vi "Calibration_Test.vi"() -> ()   [LabVIEW 2021]
uses:
  C:/Users/User/Documents/CB III control files/Thorlabs.MotionControl.Controls.dll
  CB III control files/Thorlabs.MotionControl.Controls.dll
  C:/Users/User/Documents/CB III control files/ThorLabs.MotionControl.Benchtop.DCServoCLI.dll
  CB III control files/ThorLabs.MotionControl.Benchtop.DCServoCLI.dll
  C:/Users/User/Documents/CB III control files/ThorLabs.MotionControl.KCube.DCServoCLI.dll
  CB III control files/ThorLabs.MotionControl.KCube.DCServoCLI.dll
  C:/Users/User/Documents/CB III control files/Thorlabs.MotionControl.IntegratedStepperMotorsCLI.dll
  CB III control files/Thorlabs.MotionControl.IntegratedStepperMotorsCLI.dll
  <vilib>/Utility/file.llb/Write Delimited Spreadsheet (DBL).vi
  <vilib>/Utility/file.llb/Read Delimited Spreadsheet (DBL).vi
  Global_Stop.vi
  <vilib>/ptbypt/NI_PtbyPt.lvlib
panel:
  out "Lumedica report 2":string
  in  "saveing method 2":string(combo)="SaveQueueImages"
  out "OCT ON":bool=TRUE
  out "Lumedica report":string
  in  "saveing method":string(combo)="SaveQueueImages"
  in  "?":bool
  out "OCT imaging position":dbl[](array[numeric])
  in  "?":bool
  in  "?":bool
  out "all pilot points":dbl[][](array[numeric])
  out "X-stage Control":refnum<k24>
  out "X stage properties":refnum<k24>
  in  "LongTravelStageControl":refnum<k24>(container)
  out "Zero Position":dbl[](array[numeric])
  out "Drill-Z-stage Control":refnum<k24>
  out "OCT-Z-stage-control":refnum<k24>
  out "Y-stage Control":refnum<k24>
  out "Y-stage properties":refnum<k24>
  out "Driller-Z-stage-Properties":refnum<k24>
  out "OCT-Z stage-properites":refnum<k24>
  in  "Trajectory":dbl[][](array[numeric])
  out "Velocity":T1(graph)
  out "position":T1(graph)
  in  "Driller Z- stage":refnum<k24>(container)
  in  "Y stage":refnum<k24>(container)
  in  "OCT Z-stage":refnum<k24>(container)
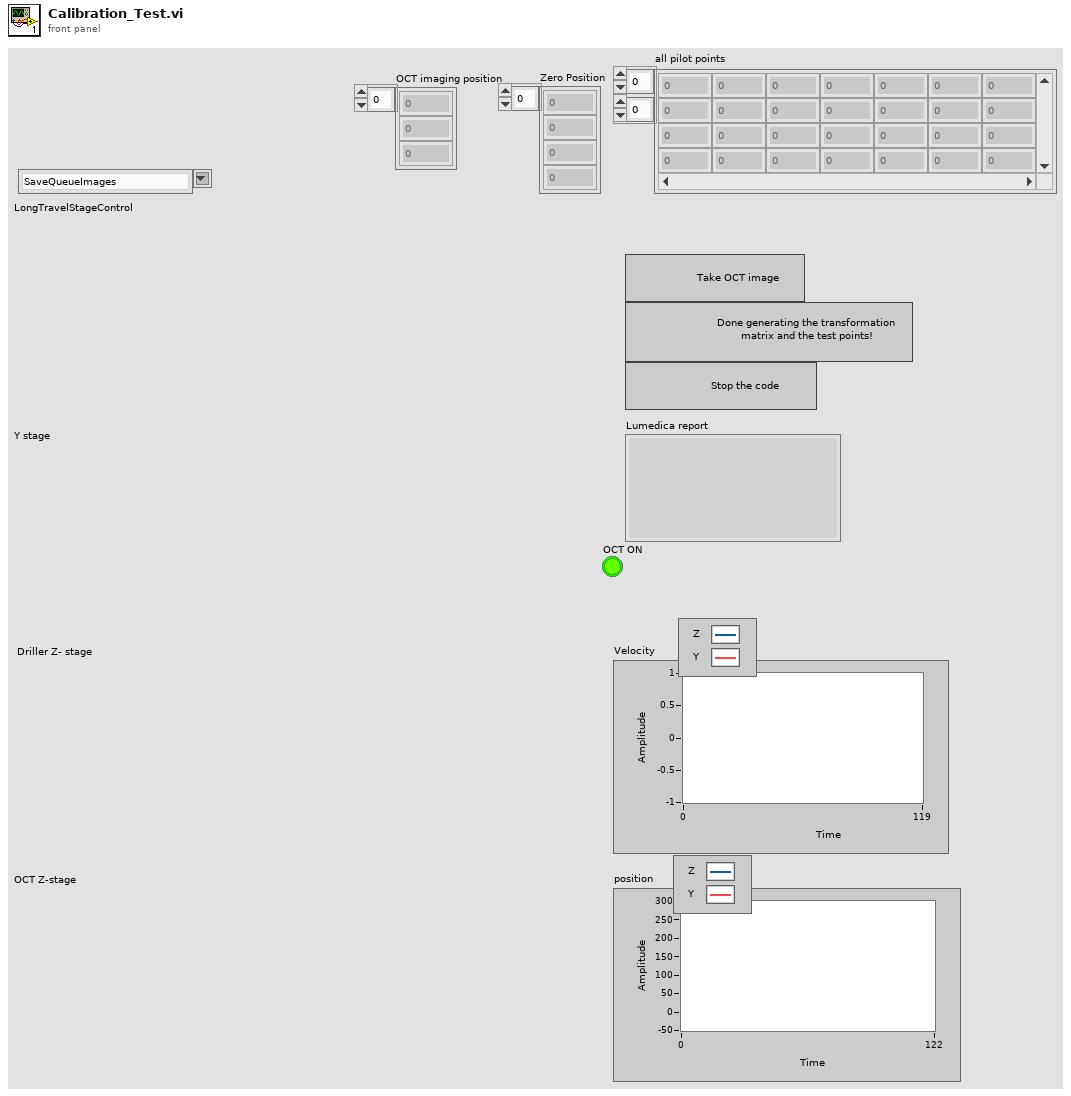
[diagram p1: front panel]
types:
  T1 = cluster{"[0]":dbl, "[1]":dbl, "[2]":dbl, "[3]":dbl, "[4]":dbl, "[5]":dbl, "[6]":dbl, "[7]":dbl, "[8]":dbl}
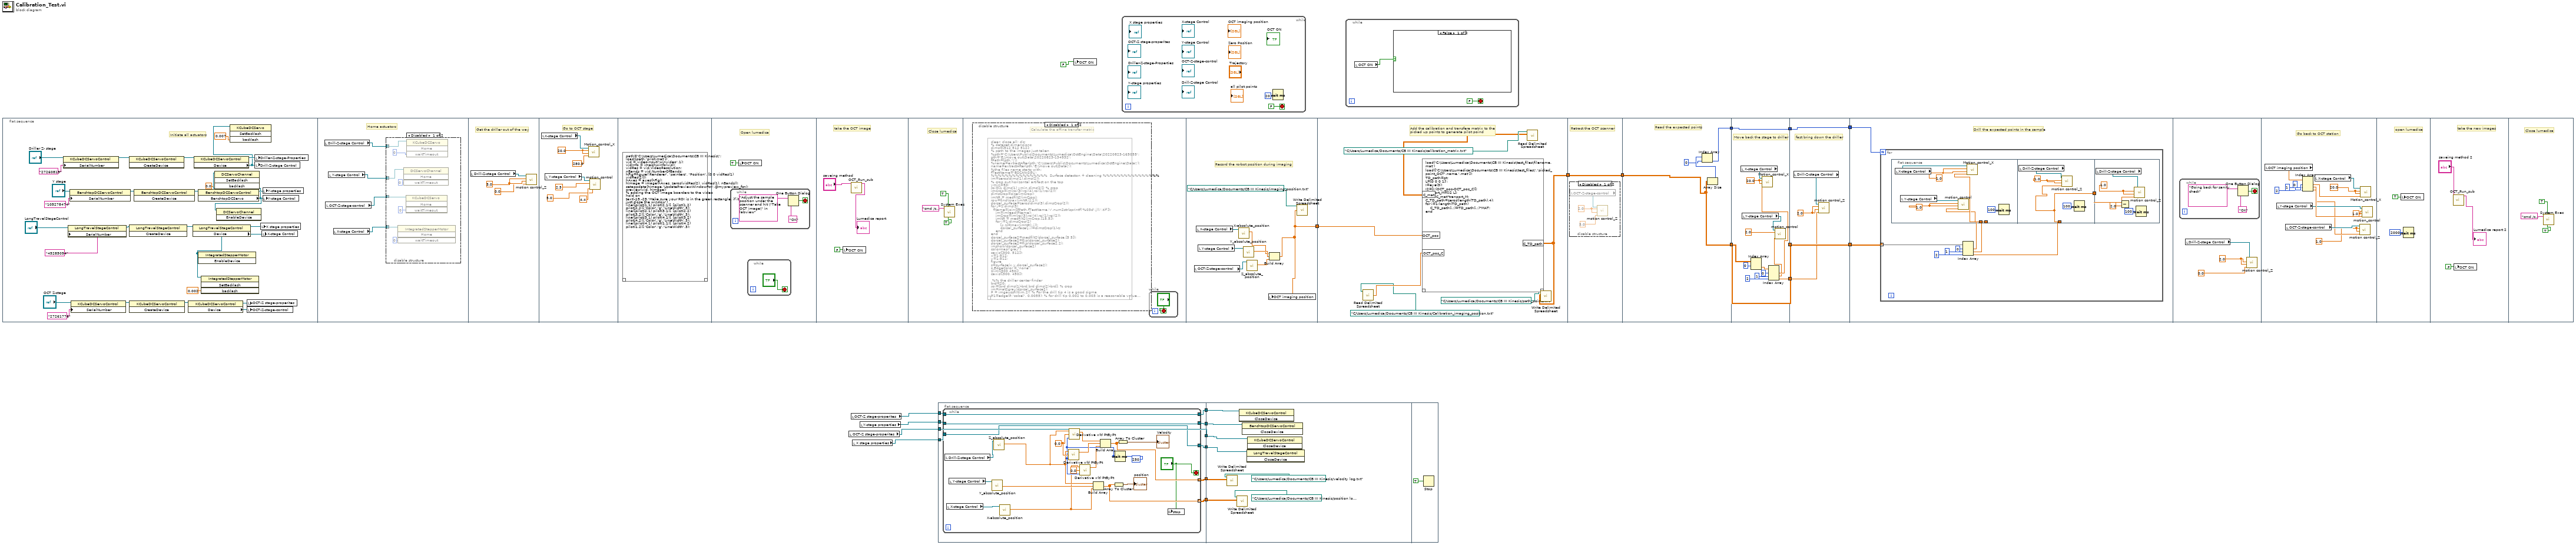
[diagram p0: block diagram]
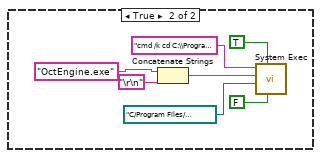
[diagram p2: hidden frame]
diagram:
  n1 = flat-sequence {
    tunnel: [w83] -> w10
    tunnel: w10 -> [w95]
    tunnel: [w91] -> w1
    tunnel: [w98] -> w2
    tunnel: w1 -> [w98]
    tunnel: [w103] -> w7
    tunnel: [w102] -> w5
    tunnel: w2 -> [w102]
    tunnel: w7 -> [w119]
    tunnel: [w119] -> w6
    tunnel: w5 -> [w114]
    tunnel: [w114] -> w4
    tunnel: [w106] -> w3
    tunnel: w6 -> [w124]
    tunnel: [w124] -> w9
    tunnel: w4 -> [w123]
    tunnel: [w123] -> w8
    tunnel: w3 -> [w120]
    tunnel: w9 -> [w126]
    tunnel: w8 -> [w125]
    frame #0 {
      # "Initiate all actuators"
      n2 = property class="KCubeDCServoControl"(reference="Driller Z- stage", "SerialNumber"="27260819") -> (reference out=w43:refnum<k24>)  [unwired: 1 in, 1 out]
      n3 = property class="LongTravelStageControl"(reference="LongTravelStageControl", "SerialNumber"="45285094") -> (reference out=w28:refnum<k24>)  [unwired: 1 in, 1 out]
      n4 = property class="BenchtopDCServoControl"(reference="Y stage", "SerialNumber"="105278474") -> (reference out=w40:refnum<k24>)  [unwired: 1 in, 1 out]
      n5 = property class="KCubeDCServoControl"(reference="OCT Z-stage", "SerialNumber"="27261776") -> (reference out=w48:refnum<k24>)  [unwired: 1 in, 1 out]
      n6 = invoke class="KCubeDCServoControl" method="CreateDevice"(reference=w43) -> (reference out=w38:refnum<k24>)  [unwired: 2 in, 2 out]
      n7 = invoke class="LongTravelStageControl" method="CreateDevice"(reference=w28) -> (reference out=w27:refnum<k24>)  [unwired: 2 in, 2 out]
      n8 = invoke class="KCubeDCServoControl" method="CreateDevice"(reference=w48) -> (reference out=w45:refnum<k24>)  [unwired: 2 in, 2 out]
      n9 = invoke class="BenchtopDCServoControl" method="CreateDevice"(reference=w40) -> (reference out=w37:refnum<k24>)  [unwired: 2 in, 2 out]
      n10 = property class="KCubeDCServoControl"(reference=w45) -> (reference out=w36:refnum<k24>, "Device"=w33:refnum<k24>)  [unwired: 1 in, 1 out]
      n11 = property class="LongTravelStageControl"(reference=w27) -> (reference out=w26:refnum<k24>, "Device"=w25:refnum<k24>)  [unwired: 1 in, 1 out]
      n12 = property class="KCubeDCServoControl"(reference=w38) -> (reference out=w35:refnum<k24>, "Device"=w31:refnum<k24>)  [unwired: 1 in, 1 out]
      n13 = property class="BenchtopDCServoControl"(reference=w37) -> (reference out=w34:refnum<k24>, "BenchtopDCServo"=w23:refnum<k24>)  [unwired: 1 in, 1 out]
      n14 = invoke class="IntegratedStepperMotor" method="EnableDevice"(reference=w25) -> ()  [unwired: 2 in, 3 out]
      n15 = invoke class="IntegratedStepperMotor" method="SetBacklash"(reference=w25, "backlash"=0.002) -> ()  [unwired: 2 in, 4 out]
      n16 = invoke class="DCServoChannel" method="SetBacklash"(reference=w23, "backlash"=0.0) -> ()  [unwired: 2 in, 4 out]
      n17 = invoke class="DCServoChannel" method="EnableDevice"(reference=w23) -> ()  [unwired: 2 in, 3 out]
      n18 = invoke class="KCubeDCServo" method="SetBacklash"(reference=w31, "backlash"=0.007) -> ()  [unwired: 2 in, 4 out]
      n19 = local write "OCT-Z stage-properites"(w36) -> ()
      n20 = local write "OCT-Z-stage-control"(w33) -> ()
      n21 = local write "Driller-Z-stage-Properties"(w35) -> ()
      n22 = local write "Drill-Z-stage Control"(w31) -> ()
      n23 = local write "X stage properties"(w26) -> ()
      n24 = local write "X-stage Control"(w25) -> ()
      n25 = local write "Y-stage properties"(w34) -> ()
      n26 = local write "Y-stage Control"(w23) -> ()
    }
    frame #1 {
      # "Home actuators"
      n27 = local read "Drill-Z-stage Control"() -> (w52:refnum<k24>)
      n28 = local read "OCT-Z-stage-control"() -> (w50:refnum<k24>)
      n29 = local read "Y-stage Control"() -> (w51:refnum<k24>)
      n30 = local read "X-stage Control"() -> (w49:refnum<k24>)
      n31 = disable-structure shown="Disabled" {
        disable-tunnel: w51 -> [w60 _]
        disable-tunnel: w52 -> [w58 _]
        disable-tunnel: w50 -> [w56 _]
        disable-tunnel: w49 -> [w54 _]
        frame Disabled {
          n32 = invoke class="IntegratedStepperMotor" method="Home"(reference=w54, "waitTimeout"=0) -> ()  [unwired: 2 in, 4 out]
          n33 = invoke class="DCServoChannel" method="Home"(reference=w60, "waitTimeout"=0) -> ()  [unwired: 2 in, 4 out]
          n34 = invoke class="KCubeDCServo" method="Home"(reference=w56, "waitTimeout"=0) -> ()  [unwired: 2 in, 4 out]
          n35 = invoke class="KCubeDCServo" method="Home"(reference=w58, "waitTimeout"=0) -> ()  [unwired: 2 in, 4 out]
        }
        frame Enabled {
        }
      }
    }
    frame #2 {
      w62 = 3.0 ("maxVelocity")
      # "Get the driller out of the way"
      n36 = local read "Drill-Z-stage Control"() -> (w63:refnum<k24>)
      n37 = call "motion control_Z.vi"("position"=0.0, "acceleration"=w62, "maxVelocity"=w62, ".NET Refnum in"=w63) -> ()  [unwired: 1 in, 1 out]
    }
    frame #3 {
      w66 = 20.0 ("maxVelocity")
      # "Go to OCT stage"
      n38 = local read "X-stage Control"() -> (w70:refnum<k24>)
      n39 = local read "Y-stage Control"() -> (w69:refnum<k24>)
      n40 = call "Motion_control_X.vi"(".NET Refnum in"=w70, "maxVelocity"=w66, "acceleration"=w66, "position"=280.0) -> ()  [unwired: 6 in, 1 out]
      n41 = call "motion_control.vi"("position"=4.4, "acceleration"=5.0, "maxVelocity"=2.5, ".NET Refnum in"=w69) -> ()  [unwired: 1 in, 1 out]
    }
    frame #4 {
      n42 = script code="path='C:\\Users\\Lumedica\\Documents\\CB III Kinesis\\';\nload([path,'pilot.mat'])\nvid = videoinput('winvideo',1);\nvidInfo = imaqhwinfo(vid);\nvidRes = vid.VideoResolution;\nnBands = vid.NumberOfBands; \nhFig=figure('Renderer', 'painters', 'Position', [0 0 vidRes(1) vidRes(2)]);\nhAxes = axes(hFig);\nhImage = image(hAxes, zeros(vidRes(2), vidRes(1), nBands)); \nsetappdata(hImage,'UpdatePreviewWindowFcn',@mypreview_fcn);\npreview(vid, hImage); \n% adding the OCT image boarders to the video\nhold on\ntext(-15,-25,'Make sure your ROI is in the green rectangle. if it is, just close the window')\nline([pilot(1,1) pilot(2,1)], [pilot(1,2) pilot(2,2)],'Color','g','LineWidth',3);\nline([pilot(2,1) pilot(3,1)], [pilot(2,2) pilot(3,2)],'Color','g','LineWidth',3);\nline([pilot(3,1) pilot(4,1)], [pilot(3,2) pilot(4,2)],'Color','g','LineWidth',3);\nline([pilot(4,1) pilot(1,1)], [pilot(4,2) pilot(1,2)],'Color','g','LineWidth',3);"() -> ()  [unwired: 1 in, 1 out]
    }
    frame #5 {
      # "Open lumedica"
      n43 = while {
        stop <- w75 stop-if-true
        n44 = One Button Dialog(message="Adjust the sample position under the scanner and hit \"Take OCT image\" in labview", button name ("OK")="OK") -> (true=w75:bool)
      }
      n45 = local write "OCT ON"(TRUE ("OCT ON")) -> ()
      n46 = while {
        stop <- "?" stop-if-true
      }
    }
    frame #6 {
      # "take the OCT image"
      n47 = local write "OCT ON"(FALSE ("OCT ON")) -> ()
      n48 = call "OCT_Run_sub.vi"("saveing method"="saveing method") -> ("Lumedica report"=→"Lumedica report":string)  [unwired: 10 in]
    }
    frame #7 {
      # "Close lumedica"
      n49 = call <vilib>:"System Exec.vi"("run minimized? (F)"=TRUE, "wait until completion? (T)"=TRUE, "command line"="cmd /c taskkill /IM OctEngine.exe") -> ()  [unwired: 5 in, 4 out]
    }
    frame #8 {
      n50 = disable-structure shown="Disabled" {
        frame Disabled {
          # "Calculate the affine transfer matrix"
          n51 = script code="clear; close all; clc;\n% dataset dimensions\ndims=[512 512 512]; \n% path to the images just taken\n%pth='C:\\Users\\Public\\Documents\\Lumedica\\OctEngine\\Data\\20220823-165055';\npth='E:\\move out\\Data\\20220823-134932';\nfPath=[pth,'\\'];\n%name=extractAfter(pth,'C:\\Users\\Public\\Documents\\Lumedica\\OctEngine\\Data\\');\nname=extractAfter(pth,'E:\\move out\\Data\\');\n%the files name starts with:\nfTestName='BSCAN-SGL';\n%%%%%%%%%%%%%%%%  Surface detecton + cleaning %%%%%%%%%%%%%%%%\nim=zeros(dims(1),dims(2)); \n% crop out horizontal artifact on the top\nymin=50;\nroi=[1 dims(1) ymin dims(2)]; % crop\nimCrop=im(roi(3):roi(4),roi(1):roi(2));\ndimsCrop=size(imCrop);\nimNR = medfilt2(imCrop);\nrow=find(max(imNR,[],1));\ndorsal_surface=zeros(dims(3),dimsCrop(2));\nfor j=1:dims(3)\n  fName=join([fPath,fTestName,'-',num2str(sprintf('%03d',j)),'.tif']);\n    im=imread(fName);\n    imCrop=im(roi(3):roi(4),roi(1):roi(2));\n    imNR = medfilt2(imCrop,[15,5]);\n    for i=1:dimsCrop(2)\n        [x,z]=max(imNR(:,i));\n        dorsal_surface(j,i)=dimsCrop(1)-z;\n    end\nend\ndorsal_surface2=medfilt2(dorsal_surface,[5 5]);\ndorsal_surface2=flip(dorsal_surface2);\ndorsal_surface2=flip(dorsal_surface2,2);\nimshow(dorsal_surface2)\ncolormap('gray')\ncaxis([300, 512]);\nx=1:512;\ny=1:512;\nfigure\ns=surface(x,y,dorsal_surface2);\ns.EdgeColor = 'none';\nzlim([300 450])\ncaxis([300, 450]);\n\n %% the driller center finder\nbrd=20;\nroi=[brd dims(1)-brd brd dims(2)-brd]; % crop\nim=mat2gray(dorsal_surface2);\nP = imgaussfilt(im,2); % For the drill tip 4 is a good sigma\nP1=edge(P,'sobel', 0.0055); % for drill tip 0.002 to 0.003 is a reasonable value\nse10 = strel('disk',2);\nP2=imdilate(P1,se10);\nP3 = imfill(P2,'holes');\nfigure\nsubplot(1,4,1)\nimshow(P1)\nsubplot(1,4,2)\nimshow(P2)\nsubplot(1,4,3)\nimshow(P3)\nP3=P3(roi(3):roi(4),roi(1):roi(2));\n[centers, radii, metric] = imfindcircles(P3,[7 45]);\ncenters=round(centers)+brd;\nsubplot(1,4,4)\n imshow(dorsal_surface2);\n caxis([300, 512]);\nviscircles(centers,radii,'LineWidth',0.4);\n% Sort the centers\ncenters=sortrows(centers,1); % right to left\ncenters=sortrows(centers,2); % sort centers top to bottom\nsave('Detected_circles5.mat','centers','radii'); \n% add their depth to them\ndorsal_surface3=medfilt2(dorsal_surface2,[5 5]);\nfor i=1:length(centers)\n    depth(i)=dorsal_surface3(centers(i,2),centers(i,1));\nend\n%% Generating the transformation matrix\n%/////////////////////DO NOT RUN DURING SANITY CHECK!\\\\\\\\\\\\\\\\\\\\\\\\\\\\\\\\\\\\\\\\\n%Generating world data\nfigure\n imshow(dorsal_surface2);\n caxis([300, 512]);\nviscircles(centers,radii,'LineWidth',0.4);\npath='C:\\Users\\User\\Documents\\CB III Kinesis\\Generated_calibration_points.txt';\npoints=importdata(path)';     %rows are each points columns are from left to right: X Y Z 1\n%Genrate OCT points in the same order\ncenters_all=[centers depth' ones(length(depth),1)];\nOCT2World=centers_all\\points; % left side multiply the transformation matrix\n[X,Y]=getpts; %press inter when done selecting\nC=[X,Y];\nfor o=1:length(X)\nviscircles([X(o),Y(o)],7.5,'LineWidth',0.4,'Color','b')\npt(o,:)=[round(X(o));round(Y(o));dorsal_surface2(round(Y(o)),round(X(o)));1]';\nW(o,:)=pt(o,:)*OCT2World;\nend\nsave(['picked_point_OCT11',name,'.mat'],'pt')\nsave(['picked_point_real',name,'.mat'],'W')\nsave(['previouse circles',name,'.mat'],'centers','radii')\nPname='C:\\Users\\User\\Documents\\CB III Kinesis\\test_points.txt';\nCLname='C:\\Users\\User\\Documents\\CB III Kinesis\\calibration_matric.txt';\nwritematrix(W,Pname,'Delimiter','tab')  % save the test point coordinates for drilling\nwritematrix(OCT2World,CLname,'Delimiter','tab') % save the calibration matrix"() -> ()  [unwired: 1 in, 1 out]
        }
        frame Enabled {
        }
      }
      n52 = while {
        stop <- "?" stop-if-true
      }
    }
    frame #9 {
      # "Record the rorbot position during imaging"
      n53 = local read "OCT-Z-stage-control"() -> (w84:refnum<k24>)
      n54 = local read "X-stage Control"() -> (w85:refnum<k24>)
      n55 = local read "Y-stage Control"() -> (w86:refnum<k24>)
      n56 = call "X-absolute_position.vi"(".NET Refnum in"=w85) -> ("Numeric"=w88:dbl)  [unwired: 9 in, 1 out]
      n57 = call "Y_absolute_position.vi"(".NET Refnum in"=w86) -> ("Numeric"=w89:dbl)  [unwired: 9 in, 1 out]
      n58 = call "Z_absolute_position.vi"(".NET Refnum in"=w84) -> ("Numeric"=w90:dbl)  [unwired: 9 in, 1 out]
      n59 = Build Array(w88, w89, w90) -> (w83:dbl[])
      n60 = local write "OCT imaging position"(w83) -> ()
      n61 = call-poly <vilib>:"Write Delimited Spreadsheet.vi"("file path (dialog if empty)"=path "C:/Users/Lumedica/Documents/CB III Kinesis/imaging_position.txt", "1D data"=w83) -> ()  [unwired: 12 in, 2 out]
    }
    frame #10 {
      # "Add the calibration and transfere matrix to the \npicked up points to generate pilot poind"
      n62 = call-poly <vilib>:"Read Delimited Spreadsheet.vi"("file path (dialog if empty)"=path "C:/Users/Lumedica/Documents/CB III Kinesis/Calibration_imaging_position.txt") -> ("first row"=w94:dbl[])  [unwired: 9 in, 5 out]
      n63 = call-poly <vilib>:"Read Delimited Spreadsheet.vi"("file path (dialog if empty)"=path "C:/Users/Lumedica/Documents/CB III Kinesis/calibration_matrix.txt") -> ("all rows"=w96:dbl[][])  [unwired: 9 in, 5 out]
      n64 = script code="load('C:\\Users\\Lumedica\\Documents\\CB III Kinesis\\test_files\\filename.mat')\nload(['C:\\Users\\Lumedica\\Documents\\CB III Kinesis\\test_files\\','picked_point_OCT',name,'.mat']);\nTD_path=pt;\nL=[0 0 0 1]';\nI=eye(3);\nI2=[I;(OCT_pos-OCT_pos_C)];\ntranport_M=[I2 L];\nMAT=C_mat*tranport_M;\nC_TD_path=zeros(length(TD_path),4);\nfor i=1:length(TD_path)\n    C_TD_path(i,:)=TD_path(i,:)*MAT;\nend"("OCT_pos_C"=w94, "OCT_pos"=w95, "C_mat"=w96) -> ("C_TD_path"=w91:dbl[][])  [unwired: 1 in, 1 out]
      n65 = call-poly <vilib>:"Write Delimited Spreadsheet.vi"("file path (dialog if empty)"=path "C:/Users/Lumedica/Documents/CB III Kinesis/path_points.txt", "2D data"=w91) -> ()  [unwired: 12 in, 2 out]
    }
    frame #11 {
      # "Retract the OCT scanner"
      n66 = disable-structure shown="Disabled" {
        frame Disabled {
          w99 = 2.0 ("maxVelocity")
          n67 = local read "OCT-Z-stage-control"() -> (w101:refnum<k24>)
          n68 = call "motion control_Z.vi"("position"=5.0, "acceleration"=w99, "maxVelocity"=w99, ".NET Refnum in"=w101) -> ()  [unwired: 1 in, 1 out]
        }
        frame Enabled {
        }
      }
    }
    frame #12 {
      # "Read the expected points"
      n69 = Array Size(array=w102) -> (size(s)=w105:i32[])
      n70 = Index Array(array=w105, index=0) -> (element=w103:i32)
    }
    frame #13 {
      w115 = 20.0 ("maxVelocity")
      w116 = 2.0 ("maxVelocity")
      # "Move back the stage to driller"
      n71 = local read "X-stage Control"() -> (w117:refnum<k24>)
      n72 = local read "Y-stage Control"() -> (w118:refnum<k24>)
      n73 = Index Array(array=w114, index (row)=0) -> (element=w112:dbl[])  [unwired: 1 in]
      n74 = Index Array(array=w112, index #1=0 ("index"), index #2=1 ("index"), index #3=2 ("index")) -> (element #1=w108:dbl, element #2=w107:dbl, element #3=w106:dbl)
      n75 = call "Motion_control_X.vi"(".NET Refnum in"=w117, "maxVelocity"=w115, "acceleration"=w115, "position"=w108) -> ()  [unwired: 6 in, 1 out]
      n76 = call "motion_control.vi"("position"=w107, "acceleration"=w116, "maxVelocity"=w116, ".NET Refnum in"=w118) -> ()  [unwired: 1 in, 1 out]
    }
    frame #14 {
      w121 = 2.0 ("acceleration")
      # "fast bring down the driller"
      n77 = local read "Drill-Z-stage Control"() -> (w122:refnum<k24>)
      n78 = call "motion control_Z.vi"("position"=w120, "acceleration"=w121, "maxVelocity"=w121, ".NET Refnum in"=w122) -> ()  [unwired: 1 in, 1 out]
    }
    frame #15 {
      # "Drill the expected points in the sample"
      n79 = for {
        N: w126 -> [_]
        tunnel: w125 -> [w134] mode=indexing
        n80 = flat-sequence {
          tunnel: w130 -> [w136]
          tunnel: w129 -> [w135]
          tunnel: w128 -> [w142]
          tunnel: [w142] -> w127
          tunnel: w127 -> [w146]
          frame #0 {
            w137 = 1.0 ("maxVelocity")
            w138 = 1.0 ("maxVelocity")
            n81 = local read "X-stage Control"() -> (w139:refnum<k24>)
            n82 = local read "Y-stage Control"() -> (w140:refnum<k24>)
            n83 = call "motion_control.vi"("position"=w135, "acceleration"=w137, "maxVelocity"=w137, ".NET Refnum in"=w140) -> ()  [unwired: 1 in, 1 out]
            n84 = call "Motion_control_X.vi"(".NET Refnum in"=w139, "maxVelocity"=w138, "acceleration"=w138, "position"=w136) -> ()  [unwired: 6 in, 1 out]
            n85 = Wait (ms)(milliseconds to wait=u32 100) -> ()  [unwired: 1 out]
          }
          frame #1 {
            w144 = 1.0 ("maxVelocity")
            n86 = local read "Drill-Z-stage Control"() -> (w145:refnum<k24>)
            n87 = call "motion control_Z.vi"("position"=w142, "acceleration"=w144, "maxVelocity"=w144, ".NET Refnum in"=w145) -> ()  [unwired: 1 in, 1 out]
            n88 = Wait (ms)(milliseconds to wait=u32 100) -> ()  [unwired: 1 out]
          }
          frame #2 {
            w150 = 1.0 ("maxVelocity")
            n89 = local read "Drill-Z-stage Control"() -> (w151:refnum<k24>)
            n90 = Subtract(x=w146, y=2.0) -> (x-y=w148:dbl)
            n91 = call "motion control_Z.vi"("position"=w148, "acceleration"=w150, "maxVelocity"=w150, ".NET Refnum in"=w151) -> ()  [unwired: 1 in, 1 out]
            n92 = Wait (ms)(milliseconds to wait=u32 100) -> ()  [unwired: 1 out]
          }
        }
        n93 = Index Array(array=w134, index #1=0 ("index"), index #2=1 ("index"), index #3=2 ("index")) -> (element #1=w130:dbl, element #2=w129:dbl, element #3=w128:dbl)
      }
    }
    frame #16 {
      w152 = 2.0 ("maxVelocity")
      n94 = while {
        stop <- w157 stop-if-true
        n95 = One Button Dialog(message="Going back for sanity check", button name ("OK")="OK") -> (true=w157:bool)
      }
      n96 = local read "Drill-Z-stage Control"() -> (w154:refnum<k24>)
      n97 = call "motion control_Z.vi"("position"=0.0, "acceleration"=w152, "maxVelocity"=w152, ".NET Refnum in"=w154) -> ()  [unwired: 1 in, 1 out]
    }
    frame #17 {
      w158 = 1.0 ("maxVelocity")
      w162 = 1.0 ("acceleration")
      w165 = 20.0 ("maxVelocity")
      # "Go back to OCT station"
      n98 = local read "OCT imaging position"() -> (w167:dbl[])
      n99 = local read "Y-stage Control"() -> (w161:refnum<k24>)
      n100 = local read "OCT-Z-stage-control"() -> (w160:refnum<k24>)
      n101 = Index Array(array=w167, index #1=0 ("index"), index #2=1 ("index"), index #3=2 ("index")) -> (element #1=w164:dbl, element #2=w163:dbl, element #3=w159:dbl)
      n102 = local read "X-stage Control"() -> (w166:refnum<k24>)
      n103 = call "motion control_Z.vi"("position"=w159, "acceleration"=w158, "maxVelocity"=w158, ".NET Refnum in"=w160) -> ()  [unwired: 1 in, 1 out]
      n104 = call "Motion_control_X.vi"(".NET Refnum in"=w166, "maxVelocity"=w165, "acceleration"=w165, "position"=w164) -> ()  [unwired: 6 in, 1 out]
      n105 = call "motion_control.vi"("position"=w163, "acceleration"=w162, "maxVelocity"=w162, ".NET Refnum in"=w161) -> ()  [unwired: 1 in, 1 out]
    }
    frame #18 {
      # "open lumedica"
      n106 = local write "OCT ON"(TRUE ("OCT ON")) -> ()
      n107 = Wait (ms)(milliseconds to wait=u32 2000) -> ()  [unwired: 1 out]
    }
    frame #19 {
      # "take the new images"
      n108 = call "OCT_Run_sub.vi"("saveing method"="saveing method 2") -> ("Lumedica report"=→"Lumedica report 2":string)  [unwired: 10 in]
      n109 = local write "OCT ON"(FALSE ("OCT ON")) -> ()
    }
    frame #20 {
      # "Close lumedica"
      n110 = call <vilib>:"System Exec.vi"("run minimized? (F)"=TRUE, "wait until completion? (T)"=TRUE, "command line"="cmd /c taskkill /IM OctEngine.exe") -> ()  [unwired: 5 in, 4 out]
    }
  }
  n111 = local read "OCT-Z stage-properites"() -> (w16:refnum<k24>)
  n112 = local read "OCT-Z stage-properites"() -> (w21:refnum<k24>)
  n113 = local read "X stage properties"() -> (w13:refnum<k24>)
  n114 = local read "Y-stage properties"() -> (w20:refnum<k24>)
  n115 = flat-sequence {
    tunnel: w21 -> [w185]
    tunnel: w20 -> [w184]
    tunnel: [w183] -> w19
    tunnel: [w187] -> w18
    tunnel: [w186] -> w17
    tunnel: w16 -> [w183]
    tunnel: [w182] -> w15
    tunnel: [w181] -> w14
    tunnel: w13 -> [w180]
    tunnel: [w179] -> w12
    tunnel: w19 -> [w213]
    tunnel: w18 -> [w214]
    tunnel: w17 -> [w215]
    tunnel: w15 -> [w211]
    tunnel: w14 -> [w209]
    tunnel: w12 -> [w208]
    frame #0 {
      n116 = while {
        tunnel: [w207] -> w187
        tunnel: w185 -> [w207]
        tunnel: w184 -> [w206]
        tunnel: [w206] -> w186
        tunnel: [w196] -> w182 mode=indexing
        tunnel: [w195] -> w181 mode=indexing
        tunnel: w180 -> [w194]
        tunnel: [w194] -> w179
        stop <- "?" stop-if-true
        w192 = u32 250 ("milliseconds to wait")
        w201 = 0.0 ("initial condition")
        n117 = local read "Drill-Z-stage Control"() -> (w197:refnum<k24>)
        n118 = local read "X-stage Control"() -> (w193:refnum<k24>)
        n119 = local read "Y-stage Control"() -> (w198:refnum<k24>)
        n120 = call "Y_absolute_position.vi"(".NET Refnum in"=w198) -> ("Numeric"=w200:dbl)  [unwired: 9 in, 1 out]
        n121 = call "Z_absolute_position.vi"(".NET Refnum in"=w197) -> ("Numeric"=w199:dbl)  [unwired: 9 in, 1 out]
        n122 = call "X-absolute_position.vi"(".NET Refnum in"=w193) -> ("Numeric"=w190:dbl)  [unwired: 9 in, 1 out]
        n123 = call <vilib>:"Derivative x(t) PtByPt.vi"("dt"=w192, "initial condition"=w201, "x"=w199) -> ("dx/dt"=w203:dbl)  [unwired: 1 in, 1 out]
        n124 = call <vilib>:"Derivative x(t) PtByPt.vi"("dt"=w192, "initial condition"=w201, "x"=w199) -> ("dx/dt"=w202:dbl)  [unwired: 1 in, 1 out]
        n125 = call <vilib>:"Derivative x(t) PtByPt.vi"("dt"=w192, "initial condition"=0.0, "x"=w190) -> ("dx/dt"=w189:dbl)  [unwired: 1 in, 1 out]
        n126 = Build Array(w199, w200, w190) -> (w195:dbl[])
        n127 = Build Array(w202, w203, w189) -> (w196:dbl[])
        n128 = Array To Cluster(array=w195) -> (cluster=→"position":T1)
        n129 = Wait (ms)(milliseconds to wait=w192) -> ()  [unwired: 1 out]
        n130 = Array To Cluster(array=w196) -> (cluster=→"Velocity":T1)
        n131 = global write "Global_Stop.vi" "stop"("?") -> ()
      }
    }
    frame #1 {
      n132 = call-poly <vilib>:"Write Delimited Spreadsheet.vi"("file path (dialog if empty)"=path "C:/Users/Lumedica/Documents/CB III Kinesis/velocity log.txt", "2D data"=w211) -> ()  [unwired: 12 in, 2 out]
      n133 = call-poly <vilib>:"Write Delimited Spreadsheet.vi"("file path (dialog if empty)"=path "C:/Users/Lumedica/Documents/CB III Kinesis/position log.txt", "2D data"=w209) -> ()  [unwired: 12 in, 2 out]
      n134 = invoke class="KCubeDCServoControl" method="CloseDevice"(reference=w214) -> ()  [unwired: 2 in, 3 out]
      n135 = invoke class="BenchtopDCServoControl" method="CloseDevice"(reference=w215) -> ()  [unwired: 2 in, 3 out]
      n136 = invoke class="LongTravelStageControl" method="CloseDevice"(reference=w208) -> ()  [unwired: 2 in, 3 out]
      n137 = invoke class="KCubeDCServoControl" method="CloseDevice"(reference=w213) -> ()  [unwired: 2 in, 3 out]
    }
    frame #2 {
      n138 = Stop(stop? (T)=TRUE) -> ()
    }
  }
  n139 = local write "OCT ON"(FALSE) -> ()
  n140 = while {
    stop <- FALSE stop-if-true
    n141 = Wait (ms)(milliseconds to wait=u32 20) -> ()  [unwired: 1 out]
  }
  n142 = while {
    stop <- FALSE stop-if-true
    n143 = local read "OCT ON"() -> (w219:bool)
    n144 = case shown="False" w219 {
      frame False {
      }
      frame True {
        n145 = Concatenate Strings("OctEngine.exe" ("string"), "\r\n") -> (w227:string)
        n146 = call <vilib>:"System Exec.vi"("run minimized? (F)"=FALSE, "wait until completion? (T)"=TRUE, "working directory"=path "C:/Program Files/Lumedica/OctEngine", "standard input"=w227, "command line"="cmd /k cd C:\\Program Files\\Lumedica\\OctEngine ") -> ()  [unwired: 3 in, 4 out]
      }
    }
  }
